vi "Resample N Waveforms (continuous, t0 DBL).vi"(0 "waveforms in":waveform(dbl)[](array[waveform]), 1 "reset":bool, 5 "dt":dbl=1.0 format="%.2p", 7 "t0":dbl=-inf format="%.2p", 9 "interpolation mode":u16(ring)=1 items=["coerce", "linear", "spline", "FIR filter"], 11 "error in (no error)":errorcluster, 12 "FIR filter specifications":T1={"alias rejection (dB)"=120.0, "normalized bandwidth"=0.4536} {"normalized bandwidth" format="%.4f"; "alias rejection (dB)" format="%.2f"}) -> (4 "resampled waveforms out":waveform(dbl)[](array[waveform]), 8 "next t0's":dbl[](array[numeric]) format="%.2p", 10 "used t0's":dbl[](array[numeric]) format="%.2p", 14 "t0 adjusted warnings":bool[](array[boolean]), 15 "error out":errorcluster)   [LabVIEW 2020, in "NI_MAPro.lvlib"]
doc: "Resamples an input waveform according to the user-defined values for <B>t0</B> and <B>dt</B>. Wire data to the <B>waveform in</B> input to determine the polymorphic instance to use or manually select the instance."
uses:
  NI_MAPro.lvlib
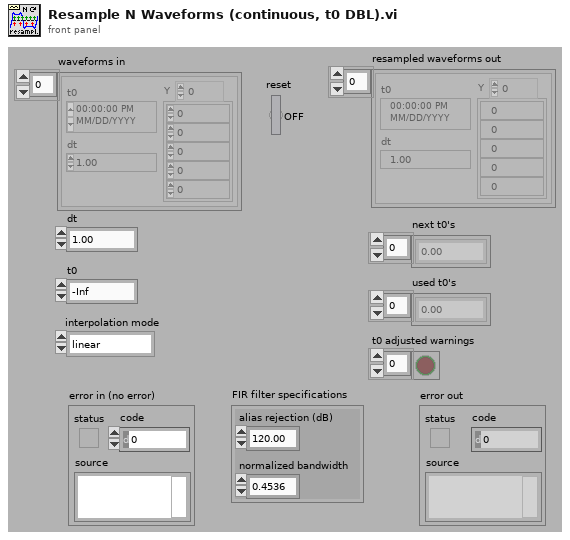
[diagram p1: front panel]
types:
  T1 = cluster{"alias rejection (dB)":dbl, "normalized bandwidth":dbl}
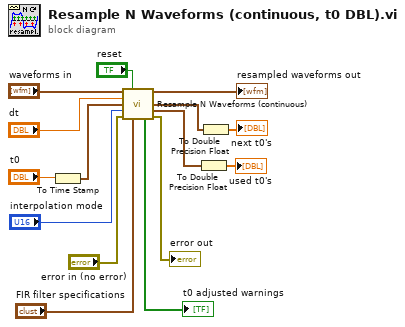
[diagram p0: block diagram]
diagram:
  n1 = To Time Stamp(1:"t0") -> (0:w3:timestamp)
  n2 = call "Resample N Waveforms (continuous).vi"("waveforms in"="waveforms in", "reset"="reset", "dt"="dt", "t0"=w3, "interpolation mode"="interpolation mode", "error in (no error)"="error in (no error)", "FIR filter specifications"="FIR filter specifications") -> ("resampled waveforms out"=→"resampled waveforms out":waveform(dbl)[], "next t0's"=w7:timestamp[], "used t0's"=w10:timestamp[], "t0 adjusted warnings"=→"t0 adjusted warnings":bool[], "error out"=→"error out":errorcluster)  [unwired: 4 in]
  n3 = To Double Precision Float(number=w10) -> (double precision float=→"used t0's":dbl[])
  n4 = To Double Precision Float(number=w7) -> (double precision float=→"next t0's":dbl[])
